vi "Create Class.vi"(8 "error in (no error)":errorcluster, 9 "Path":path, 10 "ID":string, 11 "class1 in":refnum<class "class1.lvclass">) -> (0 "error out":errorcluster, 3 "class1 out":refnum<class "class1.lvclass">)   [LabVIEW 2018, in "class1.lvclass"]
uses:
  class1.lvclass
  TypeDef/Data.ctl
  TypeDef/Settings.ctl
  class1.lvclass/class1.ctl
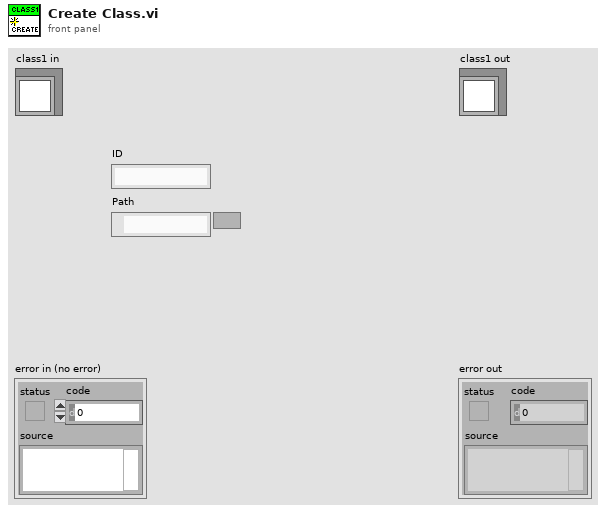
[diagram p1: front panel]
types:
  T1 = typedef "class1.lvclass/Data.ctl" = cluster{"Path":path, "ID":string, "Settings":T2, "asdf":enum16{"a", "f"}, "XY Graph":cluster{"X":dbl, "Y":dbl}[]}
  T2 = typedef "class1.lvclass/Settings.ctl" = cluster{"Speed":dbl, "Strr":string, "data":i32[]}
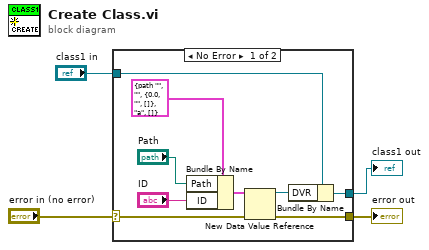
[diagram p0: block diagram]
diagram:
  n1 = case shown="No Error" "error in (no error)" {
    selector: "error in (no error)" -> [w6 w15]
    tunnel: [w5 w15] -> w3
    tunnel: [w12 w14] -> w1
    tunnel: "class1 in" -> [w13 w14]
    frame No Error {
      n2 = Bundle By Name(cluster=T1 {"Path"=path "", "ID"="", "Settings"={"Speed"=0.0, "Strr"="", "data"=[]}, "asdf"=enum."a", "XY Graph"=[]} ("Data"), "Path"="Path", "ID"="ID") -> (w11:T1)
      n3 = New Data Value Reference(data value=w11, error in=w6) -> (data value reference=w10:refnum<data-value>, error out=w5:errorcluster)
      n4 = Bundle By Name(cluster=w13, "DVR"=w10) -> (w12:refnum<class "class1.lvclass">)
    }
    frame Error {
    }
  }
  "error out" <- w3
  "class1 out" <- w1
